vi "FGVfpgaAdress.vi"(6 "ioFreqHzIn":u32=67500000 format="%.2p", 7 "Enum":T3=enum."Read", 8 "error in":errorcluster, 9 "BaseClockIn":u32=40000000 format="%.0p", 10 "FPGA VI Reference In":T2, 11 "voltageRange(+/-)In":dbl) -> (0 "error out":errorcluster, 1 "baseClockOut":u32, 2 "FPGA VI Reference Out":T2, 3 "voltageRange(+/-)Out":dbl, 4 "ioFreqHzOut":u32, 5 "Target":T1)   [LabVIEW 2016]
uses:
  controls/Enum.ctl
  controls/FPGAVIreferenceTypeDef.ctl
  controls/TargetFPGA.ctl
  <vilib>/rvi/errors/niLvFpgaAdjustHostInterfaceError.vi
  <vilib>/Utility/error.llb/Error Cluster From Error Code.vi
  <vilib>/FPGAPlugInAG/USB-7856R OEM/niLvFpga_Run_USB-7856R OEM.vi
  <vilib>/FPGAPlugInAG/USB-7856R OEM/niLvFpga_Open_USB-7856R OEM.vi
  <vilib>/rvi/interface/nirviReadWriteControl/nirviReadWriteControl.xnode
  FPGA Bitfiles/qnmController797_usbRIO_controllerFPGAmu.lvbitx
  <vilib>/rvi/interface/nirviMethod/nirviMethod.xnode
  <vilib>/rvi/interface/nirviOpenFPGA/nirviOpenFPGA.xnode
  NiFpgaLv.dll
panel:
  # "Write for the FPGA Reference has to be changed in the diagram in case need to write the adress different than RIO"
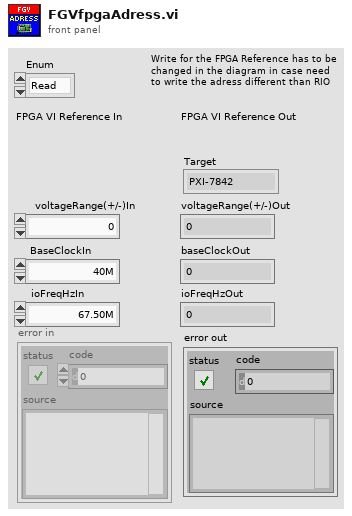
[diagram p1: front panel]
types:
  T1 = typedef "TargetFPGA.ctl" = enum16{"PXI-7842", "PXI-7851", "FlexRio-7875", "USBRio-7856R"}
  T2 = typedef "FPGAVIreferenceTypeDef.ctl" = refnum<k20>
  T3 = typedef "Enum.ctl" = enum16{"Init", "Read", "Write"}
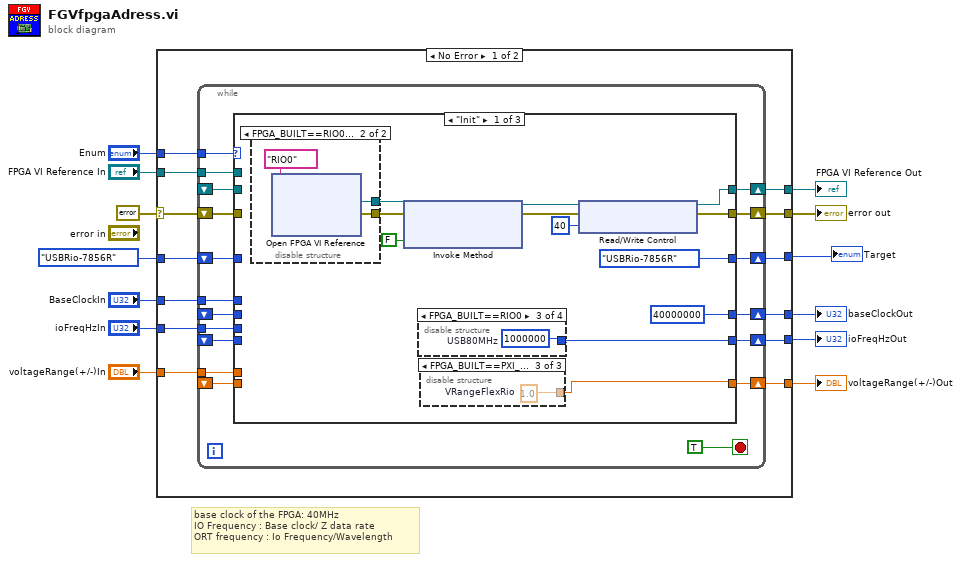
[diagram p0: block diagram]
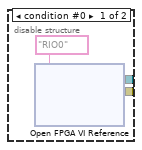
[diagram p2: hidden frame]
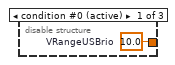
[diagram p3: hidden frame]
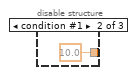
[diagram p4: hidden frame]
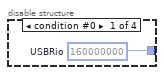
[diagram p5: hidden frame]
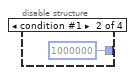
[diagram p6: hidden frame]
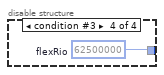
[diagram p7: hidden frame]
diagram:
  # "base clock of the FPGA: 40MHz\nIO Frequency : Base clock/ Z data rate\nORT frequency : Io Frequency/Wavelength"
  n1 = case shown="No Error" errorcluster {"status"=FALSE, "code"=0, "source"=""} ("error IO") {
    selector: errorcluster {"status"=FALSE, "code"=0, "source"=""} ("error IO") -> [w23 w87]
    tunnel: "Enum" -> [w26 _]
    tunnel: [w25 w85] -> w7
    tunnel: "FPGA VI Reference In" -> [w24 w85]
    tunnel: [w22 w87] -> w12
    tunnel: "BaseClockIn" -> [w21 w86]
    tunnel: [w20 w86] -> w11
    tunnel: "ioFreqHzIn" -> [w19 w84]
    tunnel: [w18 w84] -> w9
    tunnel: "voltageRange(+/-)In" -> [w16 w83]
    tunnel: [w17 w83] -> w5
    tunnel: [w15 w82] -> w2
    tunnel: TargetFPGA."USBRio-7856R" ("Target") -> [w14 w82]
    frame No Error {
      n2 = while {
        tunnel: w26 -> [w43]
        tunnel: w24 -> [w42]
        shift-right: [w41] -> w25
        shift-left: _ -> [w40]
        tunnel: w21 -> [w37]
        shift-right: [w36] -> w20
        shift-left: _ -> [w35]
        tunnel: w19 -> [w34]
        shift-right: [w33] -> w18
        shift-left: _ -> [w32]
        shift-right: [w38] -> w22
        shift-left: w23 -> [w39]
        shift-right: [w30] -> w17
        shift-left: _ -> [w31]
        tunnel: w16 -> [w29]
        shift-right: [w28] -> w15
        shift-left: w14 -> [w27]
        stop <- TRUE stop-if-true
        n3 = case shown="\"Init\"" w43 {
          tunnel: w42 -> [_ _ _]
          tunnel: [w53 w75 w79] -> w41
          tunnel: w40 -> [_ w75 w79]
          tunnel: w39 -> [_ w74 w81]
          tunnel: [w54 w74 w81] -> w38
          tunnel: w37 -> [_ _ w80]
          tunnel: [u32 40000000 ("ioFreqHzIn") w73 w80] -> w36
          tunnel: w35 -> [_ w73 _]
          tunnel: w34 -> [_ _ w78]
          tunnel: [w46 w72 w78] -> w33
          tunnel: w32 -> [_ w72 _]
          tunnel: w31 -> [_ w71 _]
          tunnel: [w45 w71 w77] -> w30
          tunnel: w29 -> [_ _ w77]
          tunnel: [TargetFPGA."USBRio-7856R" ("Target") w70 w76] -> w28
          tunnel: w27 -> [_ w70 w76]
          frame "Init" {
            n4 = disable-structure shown="FPGA_BUILT==RIO0, Default" {
              disable-tunnel: [w59 w61] -> w49
              disable-tunnel: [w58 w60] -> w48
              frame condition #0 {
                n5 = xnode "Open FPGA VI Reference"("resource name"=tag "RIO0") -> ("FPGA VI Reference Out"=w58:T2, "error out"=w59:errorcluster)  [unwired: 1 in]
              }
              frame condition #1 (active) {
                n6 = xnode "Open FPGA VI Reference"("resource name"=tag "RIO0") -> ("FPGA VI Reference Out"=w60:T2, "error out"=w61:errorcluster)  [unwired: 1 in]
              }
            }
            n7 = xnode "Invoke Method"("FPGA VI Reference In"=w48, "error in"=w49, "Wait Until Done (F)"=FALSE) -> ("FPGA VI Reference Out"=w56:T2, "error out"=w55:errorcluster)
            n8 = disable-structure shown="FPGA_BUILT==RIO0" {
              disable-tunnel: [w66 u32 1000000 ("USBRio") w68 w69] -> w46
              frame condition #0 {
                w66 = u32 160000000  # USBRio
              }
              frame condition #1 {
              }
              frame condition #2 (active) {
                w68 = u32 1000000  # USB80MHz
              }
              frame condition #3 {
                w69 = u32 62500000  # flexRio
              }
            }
            n9 = disable-structure shown="FPGA_BUILT==PXI_7975R" {
              disable-tunnel: [w63 10.0 ("VRangeUSBrio") w65] -> w45
              frame condition #0 (active) {
                w63 = 10.0  # VRangeUSBrio
              }
              frame condition #1 {
              }
              frame condition #2 {
                w65 = 1.0  # VRangeFlexRio
              }
            }
            n10 = xnode "Read/Write Control"("FPGA VI Reference In"=w56, "error in"=w55, "aio.i.slowInputRate"=u16 40 ("zDataRate")) -> ("FPGA VI Reference Out"=w53:T2, "error out"=w54:errorcluster)
          }
          frame "Read", Default {
          }
          frame "Write" {
          }
        }
      }
    }
    frame Error {
    }
  }
  "error out" <- w12
  "baseClockOut" <- w11
  "ioFreqHzOut" <- w9
  "FPGA VI Reference Out" <- w7
  "voltageRange(+/-)Out" <- w5
  "Target" <- w2
